vi "Read Log Instance.vi"(11 "Logger in":refnum<class "Logger.lvclass">) -> (2 "LoggerReference":refnum<class "LoggerReference.lvclass">, 3 "Logger out":refnum<class "Logger.lvclass">)   [LabVIEW 2020, in "Event Log.lvlib" / "Logger.lvclass"]
uses:
  Logger.lvclass
  <vilib>/gpm_packages/@cs/event-logger/Source/Composed Log/LoggerReference/LoggerReference.lvclass
  Logger.lvclass/Logger.ctl
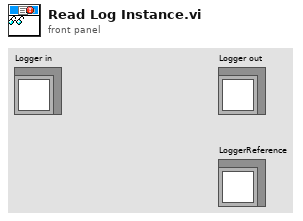
[diagram p1: front panel]
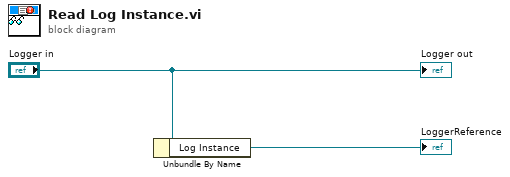
[diagram p0: block diagram]
diagram:
  n1 = Unbundle By Name("Logger in") -> ("Log Instance"=→"LoggerReference":refnum<class "LoggerReference.lvclass">)
  "Logger out" <- "Logger in"
